vi "subVI3_MAIN_checkBeforeTest_wmg.vi"(0 "input_str_SN":string) -> (1 "show_bool_checkResult":bool, 2 "show_array_failTable":string[](array[string]), 3 "show_str_failTable":string, 4 "show_messageOut":string)   [LabVIEW 2011]
uses:
  <vilib>/Utility/file.llb/Read From Spreadsheet File (string).vi
panel:
  out "show_Date":string
  out "midVar_array_tablesChnNames":string[](array[string])
  out "all rows":string[][](array[string]) caption="所有行"
  out "midVar_array_tables":string[](array[string])
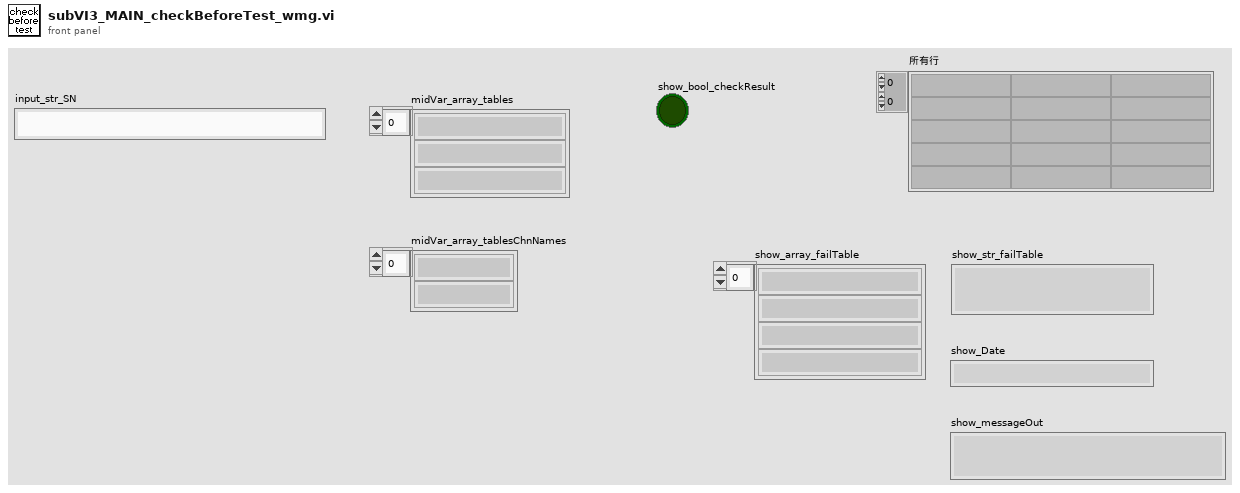
[diagram p1: front panel]
types:
  T1 = enum16{"查询表名", "查询列名", "查询记录", "查询总记录", "查询数据", "转换数据"}
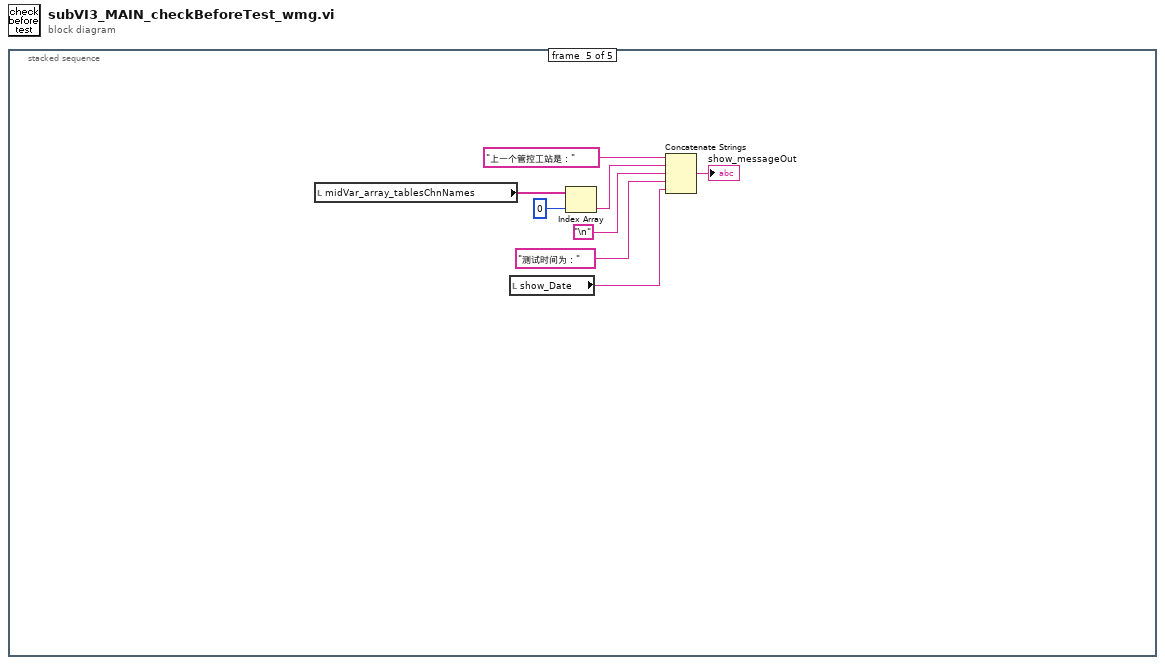
[diagram p0: block diagram]
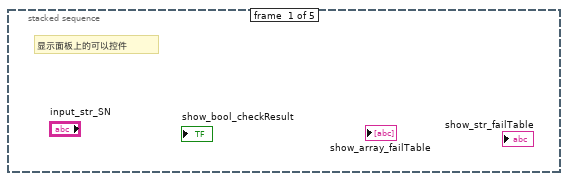
[diagram p2: hidden frame]
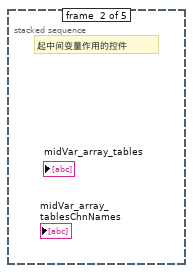
[diagram p3: hidden frame]
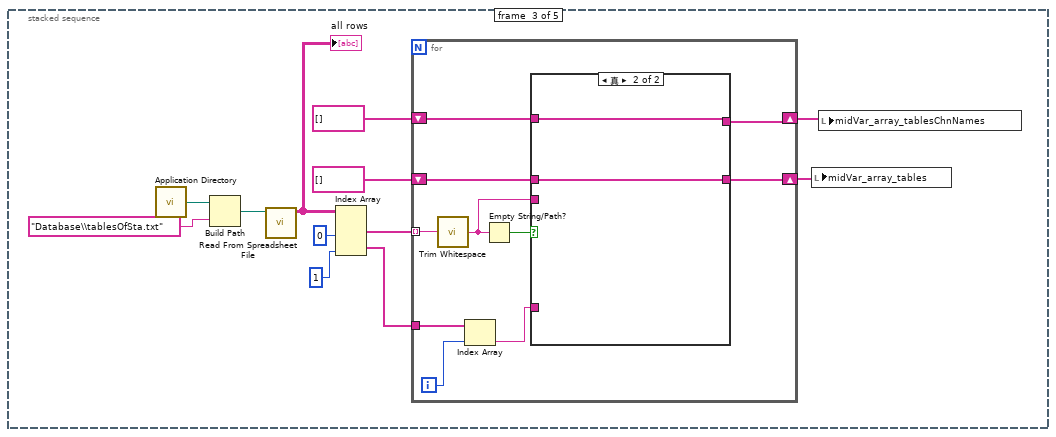
[diagram p4: hidden frame]
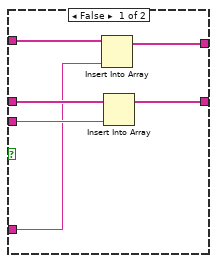
[diagram p5: hidden frame]
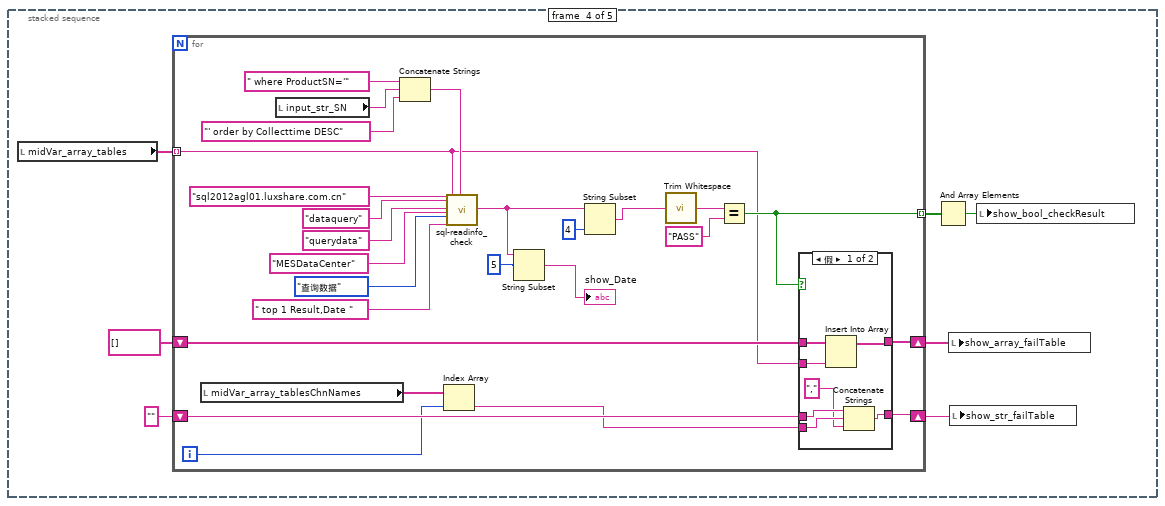
[diagram p6: hidden frame]
diagram:
  n1 = stacked-sequence {
    frame #0 {
      # "显示面板上的可以控件"
    }
    frame #1 {
      # "起中间变量作用的控件"
    }
    frame #2 {
      n2 = call <vilib>:"Application Directory.vi"() -> ("Application Directory"=w12:path)
      n3 = Build Path(base path=w12, name or relative path="Database\\tablesOfSta.txt" ("名称或相对路径")) -> (appended path=w10:path)
      n4 = call-poly <vilib>:"Read From Spreadsheet File.vi"("file path (dialog if empty)"=w10) -> ("all rows"=w9:string[][])  [unwired: 6 in, 4 out]
      "all rows" <- w9
      n5 = Index Array(array=w9, index (col) #1=0 ("禁用的索引 (列)"), index (col) #2=1 ("索引 (列)")) -> (element #1=w5:string[], element #2=w3:string[])  [unwired: 2 in]
      n6 = for {
        tunnel: w5 -> [w22] mode=indexing
        shift-right: [w18] -> w6
        shift-left: string[] [] -> [w19]
        tunnel: w3 -> [w17]
        shift-right: [w14] -> w1
        shift-left: string[] [] -> [w15]
        i -> [w16]
        n7 = call <vilib>:"Trim Whitespace.vi"("string"=w22) -> ("trimmed string"=w20:string)  [unwired: 1 in]
        n8 = Index Array(array=w17, index=w16) -> (element=w13:string)
        n9 = Empty String/Path?(string/path=w20) -> (empty?=w21:bool)
        n10 = case shown="真" w21 {
          tunnel: w20 -> [w27 _]
          tunnel: w19 -> [w28 w30]
          tunnel: [w26 w30] -> w18
          tunnel: w15 -> [w25 w29]
          tunnel: [w24 w29] -> w14
          tunnel: w13 -> [w23 _]
          frame False {
            n11 = Insert Into Array(array=w25, new element=w23) -> (w24:string[])  [unwired: 1 in]
            n12 = Insert Into Array(array=w28, new element=w27) -> (w26:string[])  [unwired: 1 in]
          }
          frame True {
          }
        }
      }
      n13 = local write "midVar_array_tables"(w6) -> ()
      n14 = local write "midVar_array_tablesChnNames"(w1) -> ()
    }
    frame #3 {
      n15 = local read "midVar_array_tables"() -> (w37:string[])
      n16 = for {
        tunnel: w37 -> [w46] mode=indexing
        tunnel: [w51] -> w36 mode=indexing
        shift-right: [w49] -> w33
        shift-left: string[] [] -> [w50]
        shift-right: [w47] -> w31
        shift-left: "" -> [w48]
        i -> [w44]
        n17 = local read "midVar_array_tablesChnNames"() -> (w45:string[])
        n18 = local read "input_str_SN"() -> (w56:string)
        n19 = Concatenate Strings(" where ProductSN='", w56, "' order by Collecttime DESC") -> (w54:string)
        n20 = Index Array(array=w45, index=w44) -> (element=w43:string)
        n21 = call "sql-readinfo_check.vi"("input-IP"="sql2012agl01.luxshare.com.cn", "input-user"="dataquery", "input-psw"="querydata", "input-db"="MESDataCenter", "操作模式"=T1."查询数据", "查询项目"=" top 1 Result,Date ", "表名"=w46, "限定条件"=w54) -> ("ResultString"=w40:string)  [unwired: 9 in, 10 out]
        n22 = String Subset(string=w40, offset (0)=5 ("长度（剩余）")) -> (substring=→"show_Date":string)  [unwired: 1 in]
        n23 = String Subset(string=w40, length (rest)=4 ("长度（剩余）")) -> (substring=w41:string)  [unwired: 1 in]
        n24 = call <vilib>:"Trim Whitespace.vi"("string"=w41) -> ("trimmed string"=w53:string)  [unwired: 1 in]
        n25 = Equal?(x=w53, y="PASS") -> (x = y?=w51:bool)
        n26 = case shown="假" w51 {
          tunnel: w50 -> [w70 w72]
          tunnel: [w69 w72] -> w49
          tunnel: w46 -> [w68 _]
          tunnel: w48 -> [w66 w71]
          tunnel: [w67 w71] -> w47
          tunnel: w43 -> [w65 _]
          frame False {
            n27 = Insert Into Array(array=w70, new element=w68) -> (w69:string[])  [unwired: 1 in]
            n28 = Concatenate Strings(w66, w65, "," ("字符串")) -> (w67:string)
          }
          frame True {
          }
        }
      }
      n29 = And Array Elements(Boolean array=w36) -> (logical AND=w35:bool)
      n30 = local write "show_array_failTable"(w33) -> ()
      n31 = local write "show_str_failTable"(w31) -> ()
      n32 = local write "show_bool_checkResult"(w35) -> ()
    }
    frame #4 {
      n33 = local read "midVar_array_tablesChnNames"() -> (w80:string[])
      n34 = local read "show_Date"() -> (w74:string)
      n35 = Index Array(array=w80, index=0 ("索引")) -> (element=w77:string)
      n36 = Concatenate Strings("上一个管控工站是：" ("字符串"), w77, "\n", "测试时间为：" ("字符串"), w74) -> (→"show_messageOut":string)
    }
  }
